vi "GetCurrent.vi"(8 "error in (no error)":errorcluster, 11 "SMU in":refnum<class "SMU.lvclass">) -> (0 "error out":errorcluster, 2 "Current, A":dbl, 3 "SMU out":refnum<class "SMU.lvclass">)   [LabVIEW 2017, in "SMU.lvclass"]
uses:
  SMU.lvclass
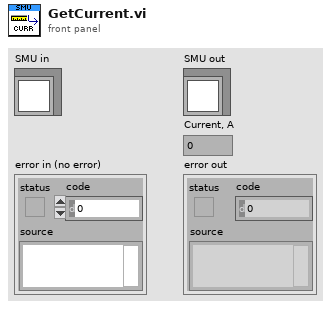
[diagram p1: front panel]
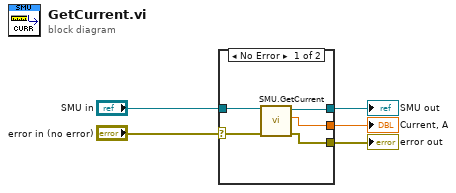
[diagram p0: block diagram]
diagram:
  n1 = case shown="No Error" "error in (no error)" {
    selector: "error in (no error)" -> [w9 w12]
    tunnel: [w8 w12] -> w4
    tunnel: [w7 w11] -> w2
    tunnel: "SMU in" -> [w10 w11]
    tunnel: [w6 _] -> w1
    frame No Error {
      n2 = call-dynamic "SMU.GetCurrent.vi"("error in (no error)"=w9, "SMU in"=w10) -> ("error out"=w8:errorcluster, "Current, A"=w6:dbl, "SMU out"=w7:refnum<class "SMU.lvclass">)  [unwired: 7 in]
    }
    frame Error {
    }
  }
  "error out" <- w4
  "SMU out" <- w2
  "Current, A" <- w1
